vi "SPCImporter_CWB.vi"(0 "start path":path=path "") -> (1 "Kaiser labels":string[](array[string]), 2 "Kaiser data":string[](array[string]), 3 "Raman labels":string[](array[string]), 4 "Raman data":string[](array[string]))   [LabVIEW 2015]
uses:
  <vilib>/Utility/error.llb/DialogType.ctl
  SPC_Folder_Convert_to_ASCII.llb/Strip Path Extension - Path__ogtk.vi
  SPC_Folder_Convert_to_ASCII.llb/Convert File Extension (String)__ogtk.vi
  <vilib>/Platform/storage/lvStorage.llb/_queryPropPoly.vi
  <vilib>/Platform/storage/lvStorage.llb/_queryPropString.vi
  <vilib>/Platform/storage/lvStorage.llb/_queryGenericObjects.vi
  <vilib>/Platform/storage/lvStorage.llb/_loadAllDouble.vi
  <vilib>/Platform/storage/lvStorage.llb/xStorage/xStorageSupp/ErrorOut.vi
  <vilib>/Platform/storage/Storage.llb/Get Object Info.vi
  <vilib>/Platform/storage/Storage.llb/__closeStorageFromObject.vi
  <vilib>/Utility/file.llb/Write To Spreadsheet File (string).vi
  <vilib>/Platform/storage/lvStorage.llb/xStorage/Read Data/Read Data.xnode
  <vilib>/Platform/storage/lvStorage.llb/xStorage/Close Data Storage/Close Data Storage.xnode
panel:
  out "match + rest of string":string
  out "SPECTRA Filename":string
  out "SPECTRA":cluster{dbl[], "Signal":dbl[]}(graph)
  in  "fixed pt":fxp<+,32,32> format="%b"
  out "Array":dbl[](array[numeric])
  out "data":u8 format="%b"
  out "EndX":dbl format="%.5g"
  out "startX":dbl format="%.5g"
  out "fnpts":u32
  out "data 3":u8 format="%x"
  out "data 2":u8 format="%x"
  out "exponent":i8
  in  "byte order (0:big-endian, network order)":T1(ring)=enum."little-endian"
  # "** Instructions: Mouse-click White Run Arrow in Toolbar and when prompted, \nSelect the Folder where the SPC files are located that you wish to convert to paired XY Ascii format**"
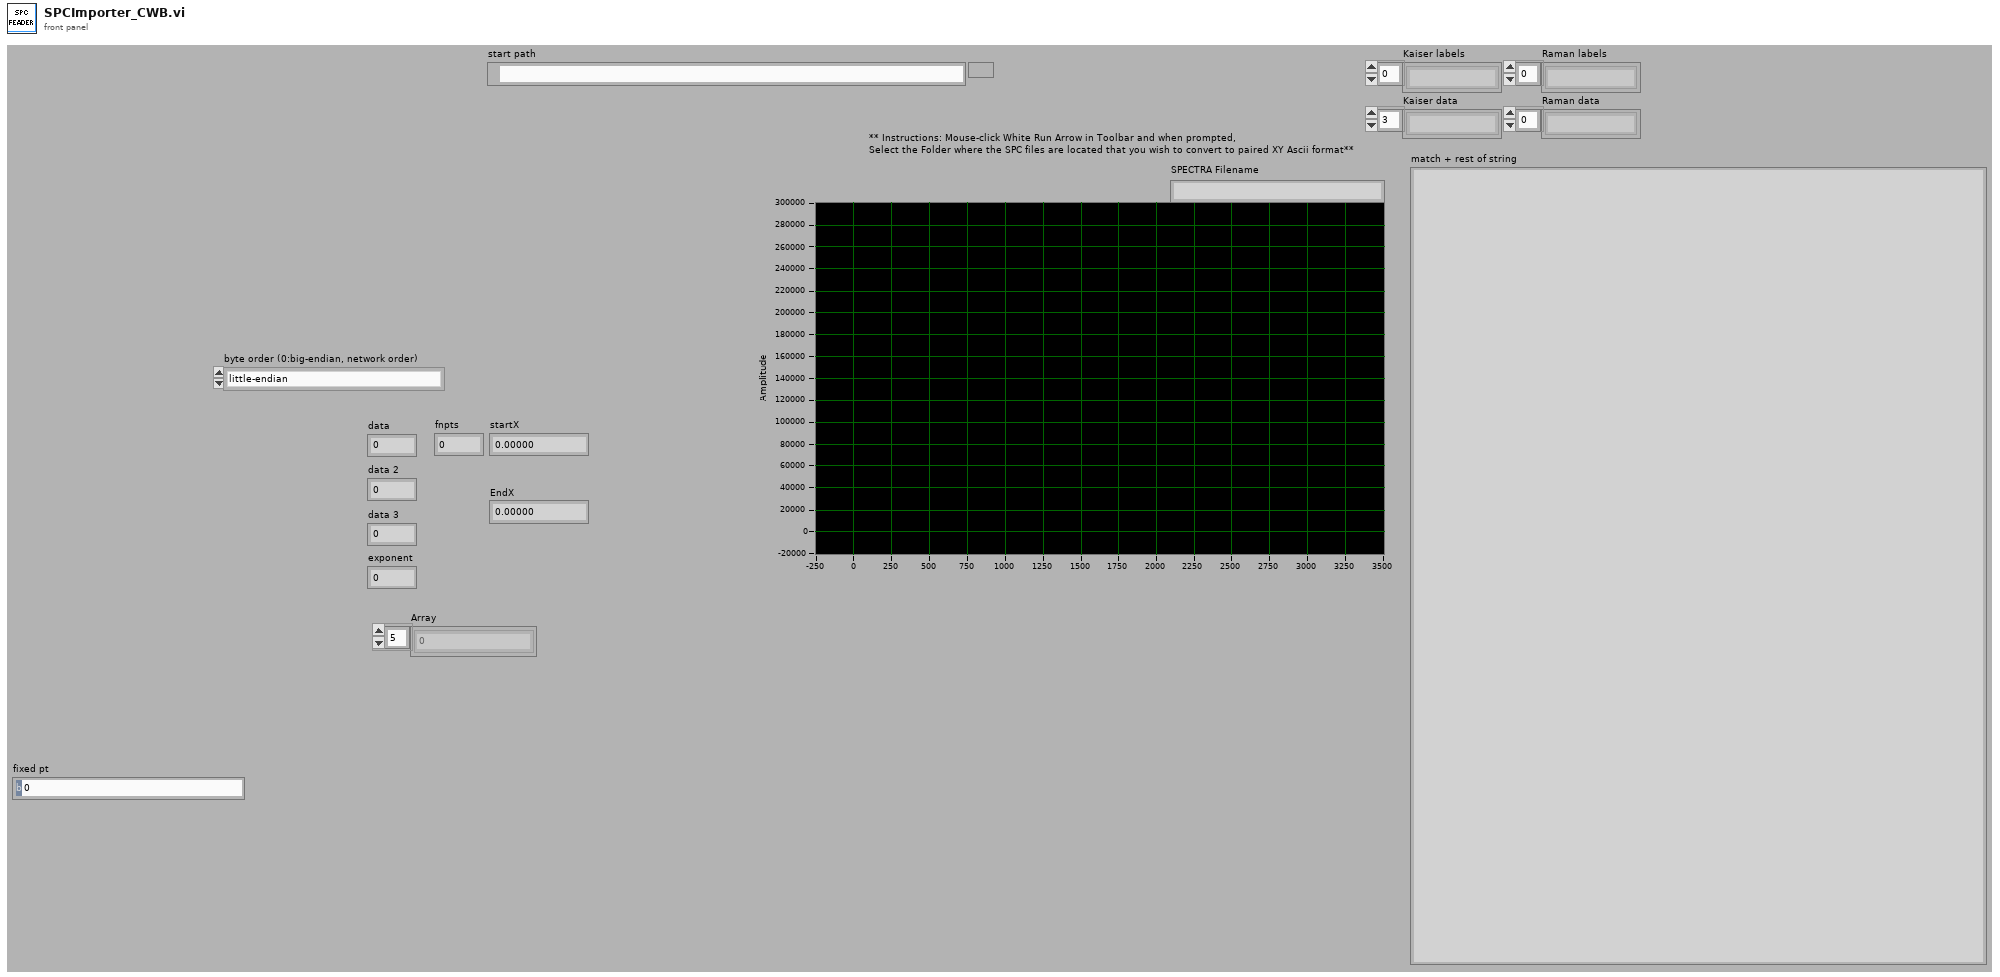
[diagram p1: front panel]
types:
  T1 = enum16{"big-endian, network order", "native, host order", "little-endian"}
  T2 = typedef "DialogType.ctl" = u16
  T3 = cluster{"fexp(I8)":i8, "fnpts(U32)":u32, "ffirst(dbl)":dbl, "flast(dbl)":dbl}
  T4 = enum16{"UPDATE", "READ", "QUERY", "CREATE CHILD", "CREATE", "CONNECT", "DISCONNECT"}
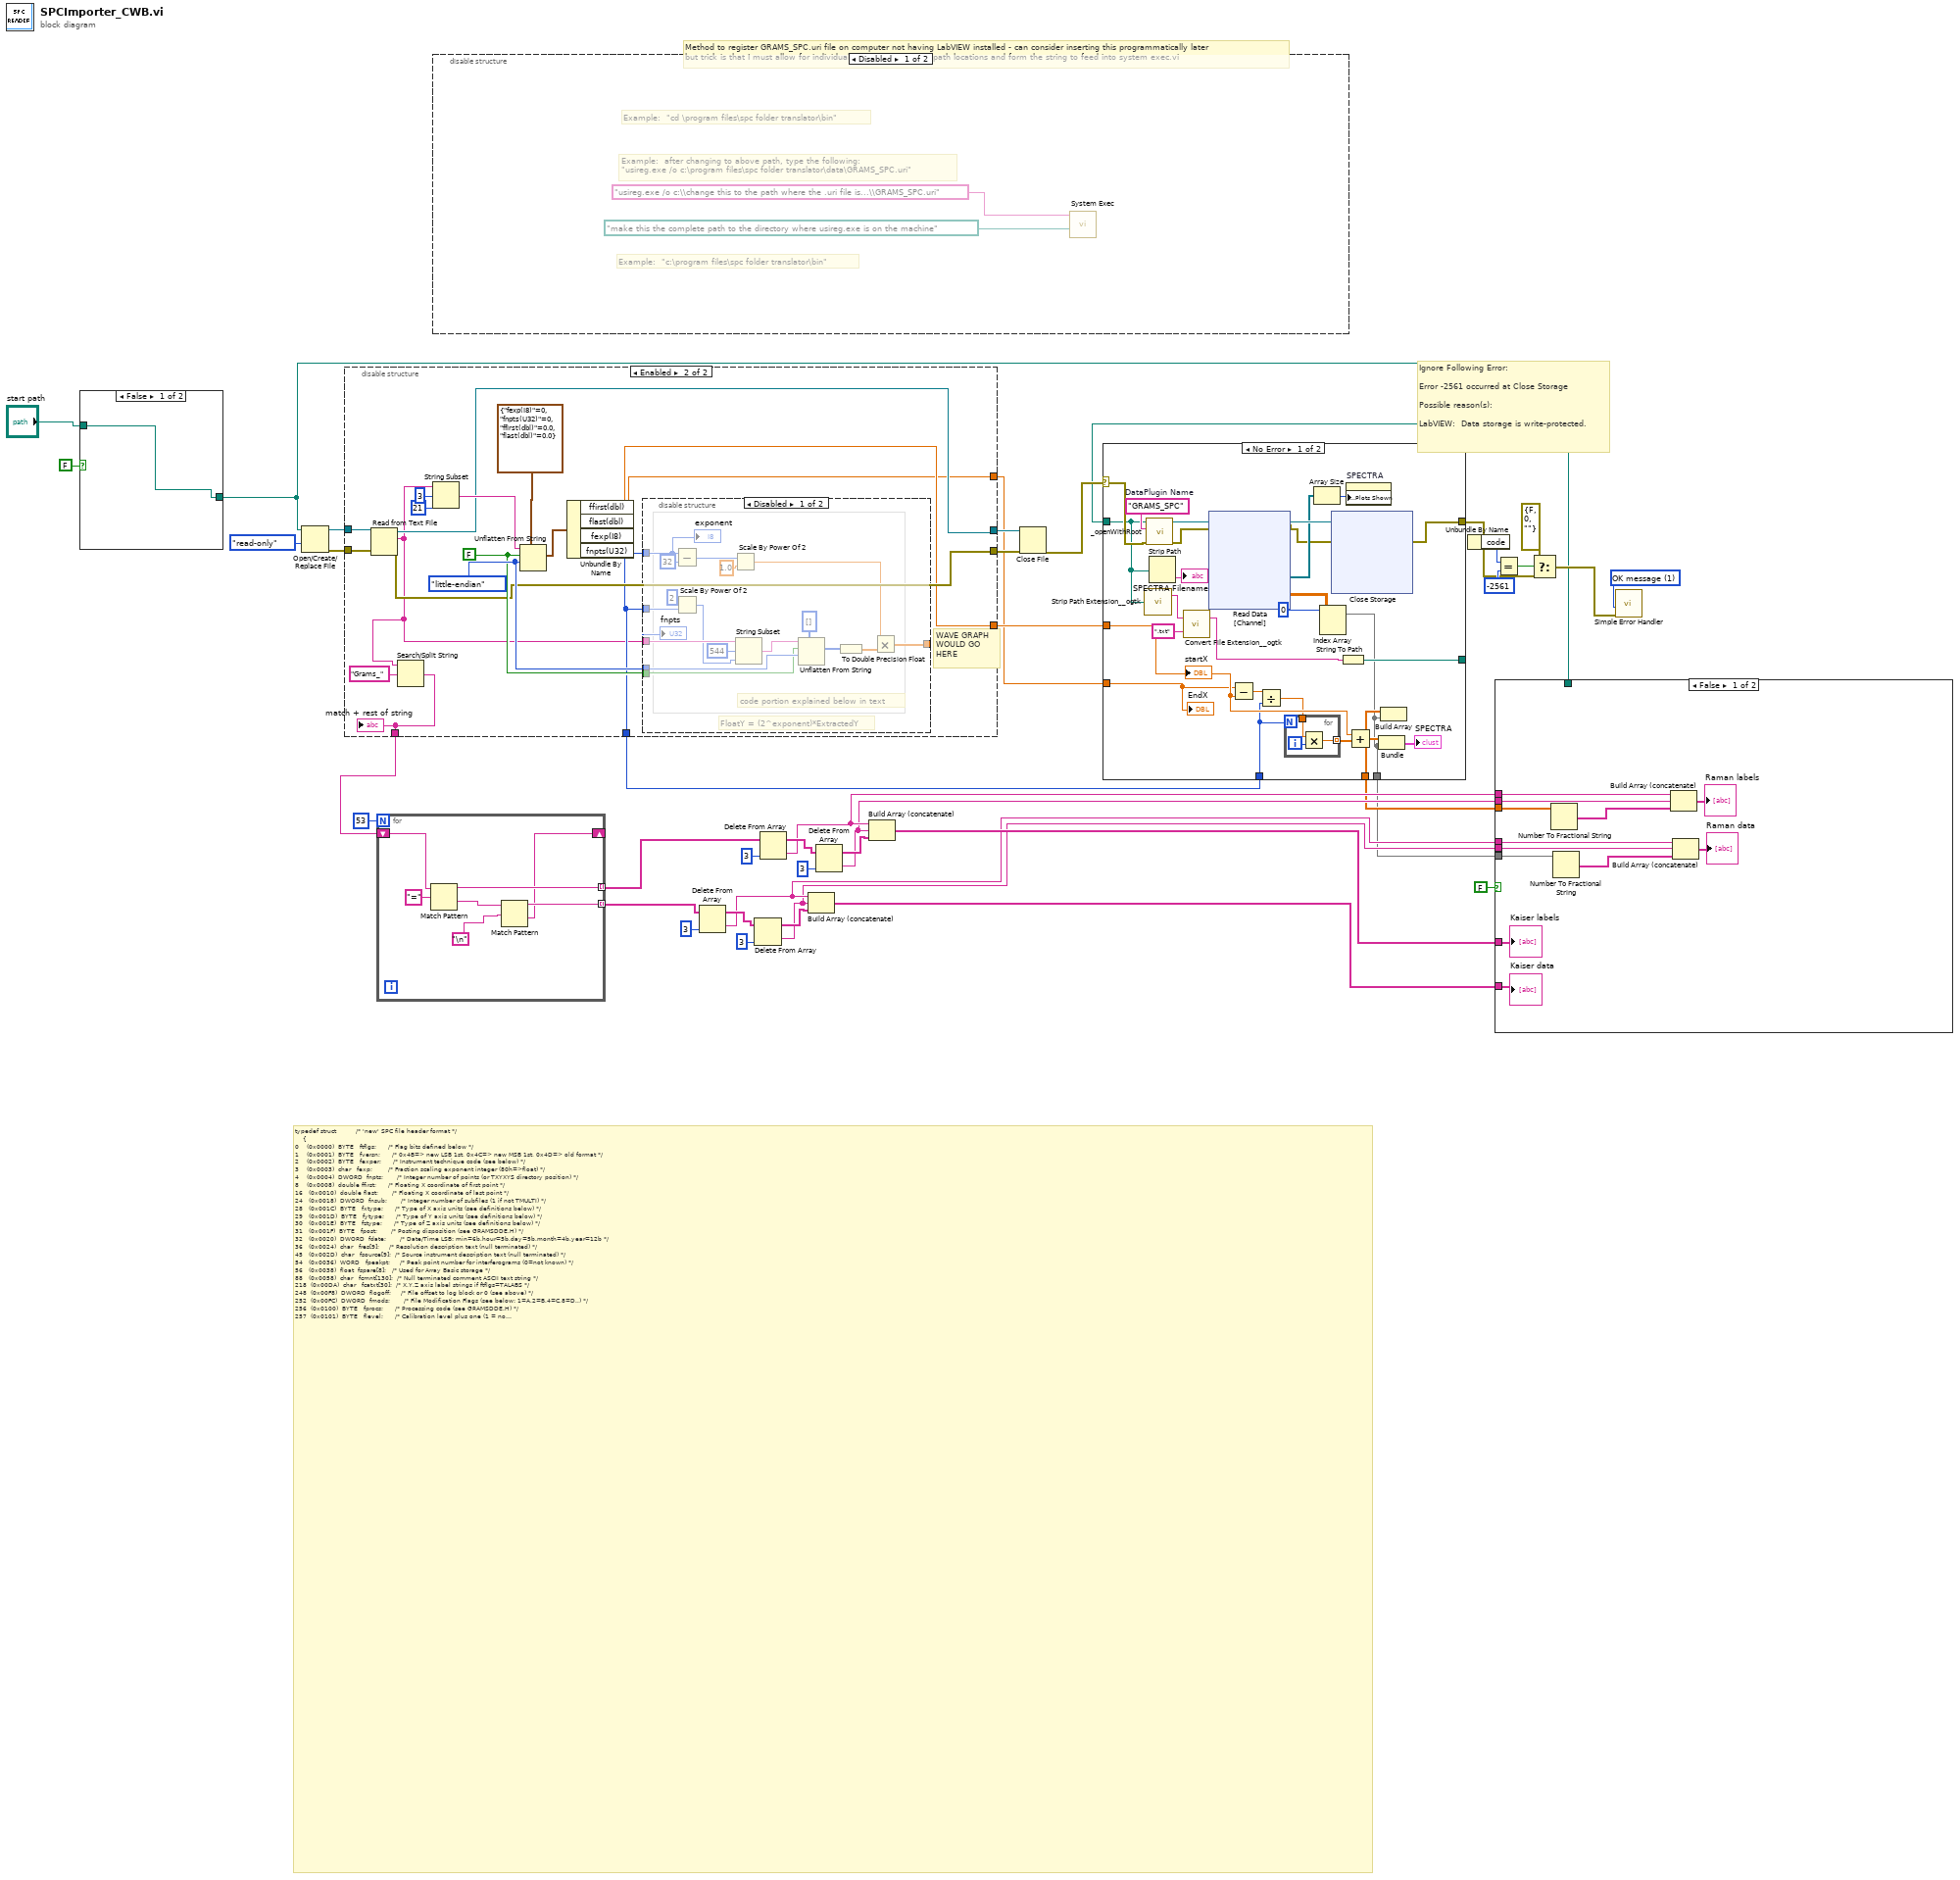
[diagram p0: block diagram]
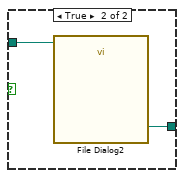
[diagram p2: hidden frame]
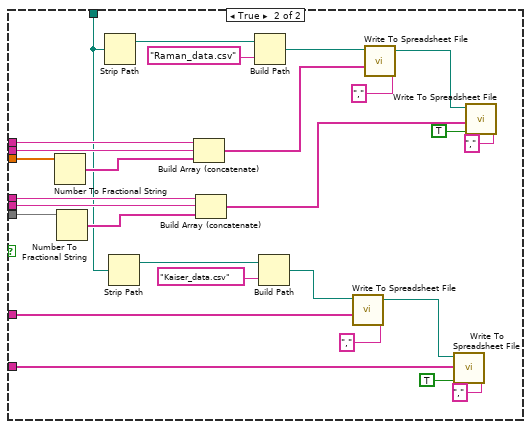
[diagram p3: hidden frame]
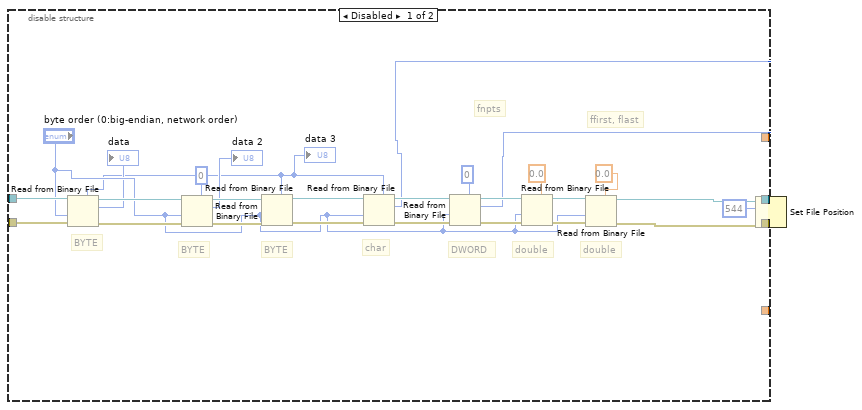
[diagram p5: hidden frame]
diagram:
  w39 = T2 1 items=["no dialog", "OK message", "continue or stop message", "OK message + warnings", "continue/stop + warnings"] ("type of dialog (OK msg:1)")
  # "Ignore Following Error:\n\nError -2561 occurred at Close Storage\n\nPossible reason(s):\n\nLabVIEW:  Data storage is write-protected."
  # "Method to register GRAMS_SPC.uri file on computer not having LabVIEW installed - can consider inserting this programmatically later\nbut trick is that I must allow for individual users to specify the path locations and form the string to feed into system exec.vi"
  # "typedef struct          /* 'new' SPC file header format */\n    {\n0    (0x0000)  BYTE   ftflgs;      /* Flag bits defined below */\n1    (0x0001)  BYTE   fversn;      /* 0x4B=> new LSB 1st, 0x4C=> new MSB 1st, 0x4D=> old format */\n2    (0x0002)  BYTE   fexper;      /* Instrument technique code (see below) */\n3    (0x0003)  char   fexp;        /* Fraction scaling exponent integer (80h=>float) */\n4    (0x0004)  DWORD  fnpts;       /* Integer number of points (or TXYXYS directory position) */\n8    (0x0008)  double ffirst;      /* Floating X coordinate of first point */\n16   (0x0010)  double flast;       /* Floating X coordinate of last point */\n24   (0x0018)  DWORD  fnsub;       /* Integer number of subfiles (1 if not TMULTI) */\n28   (0x001C)  BYTE   fxtype;      /* Type of X axis units (see definitions below) */\n29   (0x001D)  BYTE   fytype;      /* Type of Y axis units (see definitions below) */\n30   (0x001E)  BYTE   fztype;      /* Type of Z axis units (see definitions below) */\n31   (0x001F)  BYTE   fpost;       /* Posting disposition (see GRAMSDDE.H) */\n32   (0x0020)  DWORD  fdate;       /* Date/Time LSB: min=6b,hour=5b,day=5b,month=4b,year=12b */\n36   (0x0024)  char   fres[9];     /* Resolution description text (null terminated) */\n45   (0x002D)  char   fsource[9];  /* Source instrument description text (null terminated) */\n54   (0x0036)  WORD   fpeakpt;     /* Peak point number for interferograms (0=not known) */\n56   (0x0038)  float  fspare[8];   /* Used for Array Basic storage */\n88   (0x0058)  char   fcmnt[130];  /* Null terminated comment ASCII text string */\n218  (0x00DA)  char   fcatxt[30];  /* X,Y,Z axis label strings if ftflgs=TALABS */\n248  (0x00F8)  DWORD  flogoff;     /* File offset to log block or 0 (see above) */\n252  (0x00FC)  DWORD  fmods;       /* File Modification Flags (see below: 1=A,2=B,4=C,8=D..) */\n256  (0x0100)  BYTE   fprocs;      /* Processing code (see GRAMSDDE.H) */\n257  (0x0101)  BYTE   flevel;      /* Calibration level plus one (1 = not calibration data) */\n258  (0x0102)  WORD   fsampin;     /* Sub-method sample injection number (1 = first or only ) */\n260  (0x0104)  float  ffactor;     /* Floating data multiplier concentration factor (IEEE-32) */\n264  (0x0108)  char   fmethod[48]; /* Method/program/data filename w/extensions comma list */\n312  (0x0138)  float  fzinc;       /* Z subfile increment (0 = use 1st subnext-subfirst) */\n316  (0x013C)  DWORD  fwplanes;    /* Number of planes for 4D with W dimension (0=normal) */\n320  (0x0140)  float  fwinc;       /* W plane increment (only if fwplanes is not 0) */\n324  (0x0144)  BYTE   fwtype;      /* Type of W axis units (see definitions below) */\n325  (0x0145)  char   fverstr[5];  /* Extended Version identifier */\n330  (0x014A)  BYTE   fvermajor;   /* Extended Version Major revision number */\n331  (0x014B)  BYTE   fverminor;   /* Extended Version Minor revision number */\n332  (0x014C)  BYTE   finteg[20];  /* Calculated integrity value */\n352  (0x0160)  char   freserv[160];   /* Reserved (must be set to zero) */\n512  (0x0200) } SPCHDR;\n________________________________________\nDonRoth wrote:\nOn your code regarding reading the data stream (don't worry about the header), can you explain this small portion to me in greater detail so\nI understand why you did what you did? \n \n________________________________________\nAltenbach: Well, we need to read the data as little endian I32, but this will need to be divided by 2^32 and multiplied by 2^exponent. This is the same as multiplying by 2^(exponent-32).\n \nHere you need to be careful to make sure that you do this in a signed integer datatype. If you would use unsigned integers, the subtraction would lead to a huge number (because it is actually negative) and would result in a multiplier of Inf.\n \nThe upper left corner reads the exponent and subtracts 32, then calculates 1 * 2^(results if subtraction). This is the final multiplier for the data.\n \nIn the lower part we take the string subset starting at position 544. We know how many I32 points we need to read from the header, so we need to read 4x more bytes.\nUsing the x2^n node is more efficient whenever we need to multiply a blue wire with an integer power of two because computationally it is just a bit shift and no fancy\nmultiply code is needed. You can equally well just multiply with 4. Same difference.  \nNow we need to unflatten the string segment containing the data as as I32 array. The type is an empty I32 array. We select little endian, because that's the byte order\nof the datafile, and we need to wire a false because the first element does NOT contain information about the array size, but the first element.\n \n\nUPDATE - THIS STRATEGY DOES NOT WORK ALL THE TIME FOR EXTRACTING THE DATA STREAM ALTHOUGH IT IS FINE FOR THE HEADER"
  n1 = case shown="False" FALSE {
    tunnel: "start path" -> [w41 w43]
    tunnel: [w41 w42] -> w3
    frame False {
    }
    frame True {
      n2 = call "File Dialog2"("start path"=w43) -> ("selected path"=w42:path)  [unwired: 11 in, 3 out]
    }
  }
  n3 = Open/Create/Replace File(file path (use dialog)=w3, access (0:read/write)=enum16{"read/write", "read-only", "write-only"}."read-only") -> (refnum out=w36:refnum<file>, error out=w37:errorcluster)  [unwired: 4 in, 1 out]
  n4 = disable-structure shown="Enabled" {
    disable-tunnel: w37 -> [w76 w104]
    disable-tunnel: w36 -> [w75 w105]
    disable-tunnel: [w54 w95] -> w35
    disable-tunnel: [w53 w96] -> w34
    disable-tunnel: [_ w93] -> w33
    disable-tunnel: [_ w92] -> w32
    disable-tunnel: [_ w91] -> w31
    disable-tunnel: [_ w88] -> w24
    frame Disabled {
      w45 = u8 0
      # "double"
      # "double"
      # "DWORD"
      # "char"
      # "BYTE"
      # "BYTE"
      # "BYTE"
      # "ffirst, flast"
      # "fnpts"
      n5 = Read from Binary File(5:w45, 8:w76, 9:"byte order (0:big-endian, network order)", 11:w75) -> (0:w73:errorcluster, 2:→"data":u8, 3:w74:refnum<file>)  [unwired: 2 in, 1 out]
      n6 = Read from Binary File(5:w45, 8:w73, 9:"byte order (0:big-endian, network order)", 11:w74) -> (0:w71:errorcluster, 2:→"data 2":u8, 3:w72:refnum<file>)  [unwired: 2 in, 1 out]
      n7 = Read from Binary File(5:w45, 8:w71, 9:"byte order (0:big-endian, network order)", 11:w72) -> (0:w69:errorcluster, 3:w70:refnum<file>)  [unwired: 2 in, 2 out]
      n8 = Read from Binary File(5:w45, 8:w69, 9:"byte order (0:big-endian, network order)", 11:w70) -> (0:w67:errorcluster, 2:w50:u8, 3:w68:refnum<file>)  [unwired: 2 in, 1 out]
      n9 = Read from Binary File(5:u32 0, 8:w67, 9:"byte order (0:big-endian, network order)", 11:w68) -> (0:w65:errorcluster, 2:w52:u32, 3:w66:refnum<file>)  [unwired: 2 in, 1 out]
      n10 = Read from Binary File(5:0.0, 8:w65, 9:"byte order (0:big-endian, network order)", 11:w66) -> (0:w63:errorcluster, 2:w59:dbl, 3:w62:refnum<file>)  [unwired: 2 in, 1 out]
      n11 = Read from Binary File(5:0.0, 8:w63, 9:"byte order (0:big-endian, network order)", 11:w62) -> (0:w46:errorcluster, 2:w58:dbl, 3:w47:refnum<file>)  [unwired: 2 in, 1 out]
      n12 = Set File Position(offset (in bytes) (0)=i64 544, refnum=w47, error in=w46) -> (refnum out=w49:refnum<file>, error out=w48:errorcluster)  [unwired: 1 in]
      n13 = for {
        N: w52 -> [_]
        shift-right: [w85] -> w54
        shift-left: w49 -> [w87]
        shift-right: [w84] -> w53
        shift-left: w48 -> [w86]
        tunnel: w50 -> [w82]
        tunnel: [w79] -> w44 mode=indexing
        n14 = Read from Binary File(5:"fixed pt", 8:w86, 11:w87) -> (0:w84:errorcluster, 2:w81:fxp<+,32,32>, 3:w85:refnum<file>)  [unwired: 3 in, 1 out]
        n15 = To Double Precision Float(number=w81) -> (double precision float=w77:dbl)
        n16 = To Double Precision Float(number=w82) -> (double precision float=w83:dbl)
        n17 = Power Of 2(x=w83) -> (2^x=w80:dbl)
        n18 = Multiply(x=w80, y=w77) -> (x*y=w79:dbl)
      }
      "Array" <- w44
      "data 3" <- w45
    }
    frame Enabled {
      w98 = T1."little-endian" ("byte order (0:big-endian, network order)")
      w97 = FALSE ("data includes array or string size? (T)")
      # "WAVE GRAPH\nWOULD GO\nHERE"
      n19 = Read from Text File(file (use dialog)=w105, error in=w104) -> (refnum out=w95:refnum<file>, text=w90:string, error out=w96:errorcluster)  [unwired: 2 in, 1 out]
      n20 = Search/Split String(string=w90, search string/char (-)="Grams_") -> (match + rest of string=w88:string)  [unwired: 1 in, 2 out]
      "match + rest of string" <- w88
      n21 = String Subset(string=w90, offset (0)=3, length (rest)=21 ("length (rest)")) -> (substring=w100:string)
      n22 = Unflatten From String(type=T3 {"fexp(I8)"=0, "fnpts(U32)"=0, "ffirst(dbl)"=0.0, "flast(dbl)"=0.0}, binary string=w100, data includes array or string size? (T)=w97, byte order (0:big-endian, network order)=w98) -> (value=w99:T3)  [unwired: 1 in, 2 out]
      n23 = Unbundle By Name(w99) -> ("ffirst(dbl)"=w93:dbl, "flast(dbl)"=w92:dbl, "fexp(I8)"=w94:i8, "fnpts(U32)"=w91:u32)
      n24 = disable-structure shown="Disabled" {
        disable-tunnel: w90 -> [w120 _]
        disable-tunnel: [w110 _] -> _
        disable-tunnel: w98 -> [w109 _]
        disable-tunnel: w97 -> [w108 _]
        disable-tunnel: w94 -> [w107 _]
        disable-tunnel: w91 -> [w106 _]
        frame Disabled {
          # "FloatY = (2^exponent)*ExtractedY"
          # "code portion explained below in text"
          n25 = Subtract(x=w107, y=i8 32) -> (x-y=w115:i8)
          n26 = Scale By Power Of 2(n=2, x=w106) -> (x*2^n=w118:u32)
          n27 = Scale By Power Of 2(n=w115, x=1.0) -> (x*2^n=w112:dbl)
          n28 = String Subset(string=w120, offset (0)=544, length (rest)=w118) -> (substring=w117:string)
          n29 = Unflatten From String(type=i32[] [], binary string=w117, data includes array or string size? (T)=w108, byte order (0:big-endian, network order)=w109) -> (value=w113:i32[])  [unwired: 1 in, 2 out]
          n30 = To Double Precision Float(number=w113) -> (double precision float=w111:dbl[])
          n31 = Multiply(x=w112, y=w111) -> (x*y=w110:dbl[])
          "exponent" <- w107
          "fnpts" <- w106
        }
        frame Enabled {
        }
      }
    }
  }
  n32 = for {
    N: 53 -> [_]
    tunnel: [w127] -> w22 mode=indexing
    tunnel: [w125] -> w13 mode=indexing
    shift-right: [w124] -> _
    shift-left: w24 -> [w128]
    n33 = Match Pattern(string=w128, regular expression="=" ("search string/char (-)")) -> (before substring=w127:string, after substring=w126:string)  [unwired: 1 in, 2 out]
    n34 = Match Pattern(string=w126, regular expression="\n") -> (before substring=w125:string, after substring=w124:string)  [unwired: 1 in, 2 out]
  }
  n35 = disable-structure shown="Disabled" {
    frame Disabled {
      # "Example:  after changing to above path, type the following:\n\"usireg.exe /o c:\\program files\\spc folder translator\\data\\GRAMS_SPC.uri\""
      # "Example:  \"c:\\program files\\spc folder translator\\bin\""
      # "Example:  \"cd \\program files\\spc folder translator\\bin\""
      n36 = call <vilib>:"System Exec.vi"("working directory"=path "make this the complete path to the directory where usireg.exe is on the machine", "command line"="usireg.exe /o c:\\change this to the path where the .uri file is...\\GRAMS_SPC.uri") -> ()  [unwired: 6 in, 4 out]
    }
    frame Enabled {
    }
  }
  n37 = Delete From Array(array=w13, index=3) -> (deleted portion=w7:string, array with subset deleted=w16:string[])  [unwired: 1 in]
  n38 = Delete From Array(array=w16, index=3) -> (deleted portion=w6:string, array with subset deleted=w14:string[])  [unwired: 1 in]
  n39 = Delete From Array(array=w22, index=3) -> (deleted portion=w10:string, array with subset deleted=w20:string[])  [unwired: 1 in]
  n40 = Build Array (concatenate)(w7, w6, w14) -> (w12:string[])
  n41 = Delete From Array(array=w20, index=3) -> (deleted portion=w9:string, array with subset deleted=w18:string[])  [unwired: 1 in]
  n42 = Build Array (concatenate)(w10, w9, w18) -> (w11:string[])
  n43 = Close File(refnum=w35, error in=w34) -> (error out=w25:errorcluster)  [unwired: 1 out]
  n44 = case shown="No Error" w25 {
    selector: w25 -> [w140 w183]
    tunnel: w3 -> [w136 _]
    tunnel: [w150 w183] -> w26
    tunnel: w33 -> [w147 _]
    tunnel: w32 -> [w146 _]
    tunnel: w31 -> [w141 _]
    tunnel: [w134 _] -> _
    tunnel: [w133 _] -> w8
    tunnel: [w132 _] -> w5
    frame No Error {
      w157 = "GRAMS_SPC"  # DataPlugin Name
      n45 = call-poly "Strip Path Extension__ogtk.vi"("path"=w136) -> ("root"=w139:string)  [unwired: 1 out]
      n46 = call <vilib>:"_openWithRoot.vi"("error in (no error)"=w140, "Storage Type"=w157, "Storage Location"=w136) -> ("error out"=w155:errorcluster, "Data object"=w156:refnum<k20>)  [unwired: 7 in]
      n47 = Strip Path(path=w136) -> (name=→"SPECTRA Filename":string)  [unwired: 1 out]
      n48 = call-poly "Convert File Extension__ogtk.vi"("new ending (none)"=".txt", "file name"=w139) -> ("new filename"=w137:string)  [unwired: 1 out]
      n49 = xnode "Read Data\n[Channel]"("storage refnum (file)"=w156, "error in"=w155) -> ("storage refnums (channel)"=w153:refnum<k20>[], "Signal"=w151:dbl[][], "storage refnum (file) out"=w154:refnum<k20>, "error out"=w149:errorcluster)
      n50 = Subtract(x=w146, y=w147) -> (x-y=w145:dbl)
      n51 = Divide(x=w145, y=w141) -> (x/y=w144:dbl)
      n52 = for {
        N: w141 -> [_]
        tunnel: w144 -> [w159]
        tunnel: [w158] -> w143 mode=indexing
        i -> [w160]
        n53 = Multiply(x=w159, y=w160) -> (x*y=w158:dbl)
      }
      n54 = Array Size(array=w153) -> (size(s)=w152:i32)
      n55 = Index Array(array=w151, index (row)=0) -> (element=w132:dbl[])  [unwired: 1 in]
      n56 = xnode "Close Storage\n"("storage refnum (file)"=w154, "error in (no error)"=w149) -> ("error out"=w150:errorcluster)  [unwired: 1 out]
      n57 = String To Path(string=w137) -> (path=w134:path)
      n58 = property on="SPECTRA" class="XYGraph (strict)"("Legend:Plots Shown"=w152) -> ()  [unwired: 2 in, 2 out]
      n59 = Add(x=w147, y=w143) -> (x+y=w133:dbl[])
      n60 = Bundle(w133, "Signal"=w132) -> (→"SPECTRA":cluster{dbl[], "Signal":dbl[]})  [unwired: 1 in]
      n61 = Build Array(w133, w132) -> ()  [unwired: 1 out]
      "startX" <- w147
      "EndX" <- w146
    }
    frame Error {
    }
  }
  n62 = Unbundle By Name(w26) -> ("code"=w30:i32)
  n63 = Equal?(x=w30, y=-2561) -> (x = y?=w28:bool)
  n64 = case shown="False" FALSE {
    tunnel: w12 -> [w186 w216]
    tunnel: w11 -> [w187 w215]
    tunnel: w10 -> [w191 w211]
    tunnel: w9 -> [w192 w210]
    tunnel: w8 -> [w193 w209]
    tunnel: w7 -> [w190 w200]
    tunnel: w6 -> [w189 w199]
    tunnel: w5 -> [w188 w198]
    tunnel: w3 -> [_ w196]
    frame False {
      n65 = Number To Fractional String(number=w193) -> (F-format string=w195:string[])  [unwired: 3 in]
      n66 = Number To Fractional String(number=w188) -> (F-format string=w194:string[])  [unwired: 3 in]
      n67 = Build Array (concatenate)(w191, w192, w195) -> (→"Raman labels":string[])
      n68 = Build Array (concatenate)(w190, w189, w194) -> (→"Raman data":string[])
      "Kaiser labels" <- w187
      "Kaiser data" <- w186
    }
    frame True {
      n69 = Number To Fractional String(number=w209) -> (F-format string=w208:string[])  [unwired: 3 in]
      n70 = Number To Fractional String(number=w198) -> (F-format string=w201:string[])  [unwired: 3 in]
      n71 = Strip Path(path=w196) -> (stripped path=w213:path)  [unwired: 1 out]
      n72 = Strip Path(path=w196) -> (stripped path=w222:path)  [unwired: 1 out]
      n73 = Build Array (concatenate)(w211, w210, w208) -> (w202:string[])
      n74 = Build Array (concatenate)(w200, w199, w201) -> (w197:string[])
      n75 = Build Path(base path=w213, name or relative path="Raman_data.csv") -> (appended path=w203:path)
      n76 = Build Path(base path=w222, name or relative path="Kaiser_data.csv") -> (appended path=w214:path)
      n77 = call-poly <vilib>:"Write To Spreadsheet File.vi"("delimiter (\\t)"="," ("delimiter (\\t)"), "1D data"=w215, "file path (dialog if empty)"=w214) -> ("new file path (Not A Path if cancelled)"=w217:path)  [unwired: 5 in]
      n78 = call-poly <vilib>:"Write To Spreadsheet File.vi"("delimiter (\\t)"="," ("delimiter (\\t)"), "1D data"=w202, "file path (dialog if empty)"=w203) -> ("new file path (Not A Path if cancelled)"=w204:path)  [unwired: 5 in]
      n79 = call-poly <vilib>:"Write To Spreadsheet File.vi"("delimiter (\\t)"="," ("delimiter (\\t)"), "append to file? (new file:F)"=TRUE, "1D data"=w216, "file path (dialog if empty)"=w217) -> ()  [unwired: 4 in, 1 out]
      n80 = call-poly <vilib>:"Write To Spreadsheet File.vi"("delimiter (\\t)"="," ("delimiter (\\t)"), "append to file? (new file:F)"=TRUE, "1D data"=w197, "file path (dialog if empty)"=w204) -> ()  [unwired: 4 in, 1 out]
    }
  }
  n81 = Select(t=errorcluster {"status"=FALSE, "code"=0, "source"=""} ("error out"), s=w28, f=w26) -> (s? t:f=w40:errorcluster)
  n82 = call <vilib>:"Simple Error Handler.vi"("type of dialog (OK msg:1)"=w39, "error in (no error)"=w40) -> ()  [unwired: 3 in, 5 out]
